vi "Generate Thetas.vi"(0 "spline flat":cluster{"x":sgl, "y":sgl}[](array[cluster]), 5 "starting angle":sgl, 7 "dt":sgl=0.02, 9 "ctrl pts":cluster{sgl, sgl}[][](array[cluster]), 11 "y unflat":cluster{dbl[]}[](array[cluster])) -> (4 "omega":sgl[](array[numeric]), 6 "theta":sgl[](array[numeric]), 10 "Tangent Vector":cluster{"x out":dbl, "y out":dbl}[](array[cluster]))   [LabVIEW 2025]
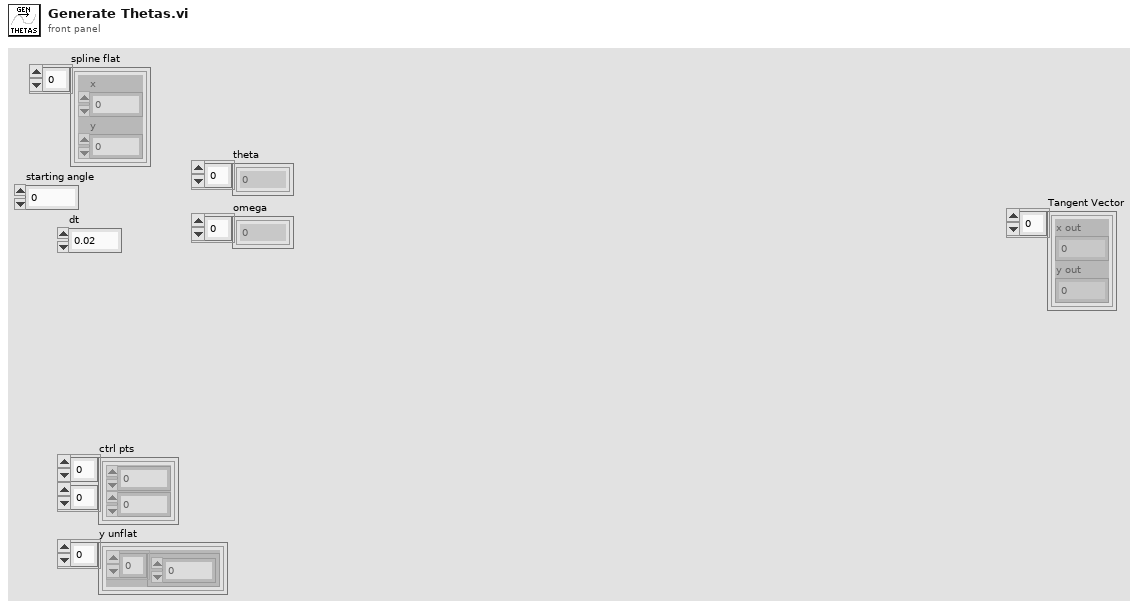
[diagram p1: front panel]
types:
  T1 = typedef "Bezier Curve.ctl" = cluster{"x":sgl, "y":sgl}[]
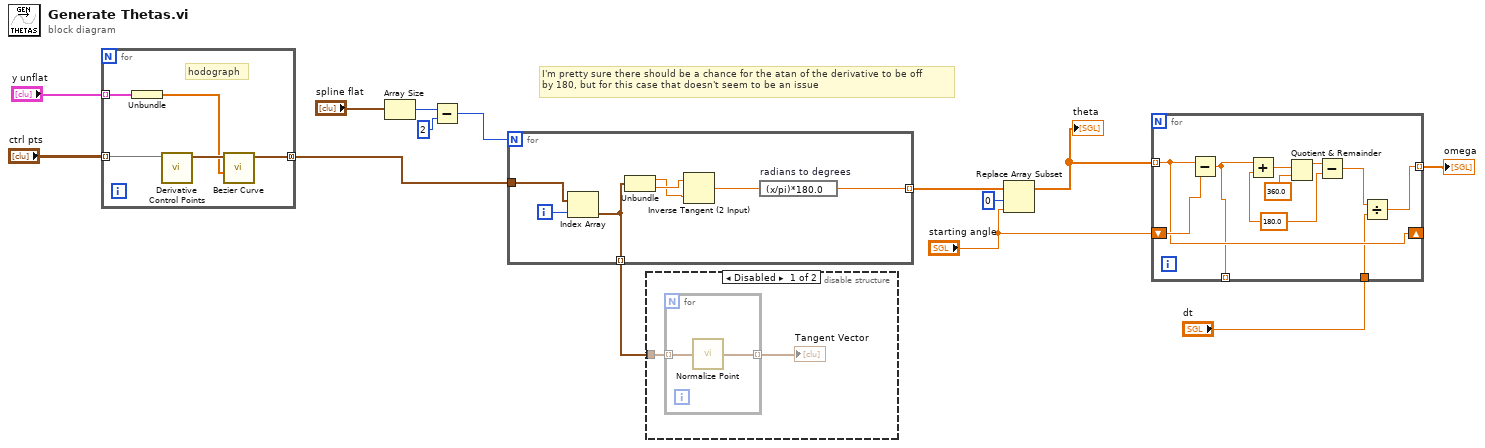
[diagram p0: block diagram]
diagram:
  # "I'm pretty sure there should be a chance for the atan of the derivative to be off\nby 180, but for this case that doesn't seem to be an issue"
  n1 = for {
    tunnel: "ctrl pts" -> [w19] mode=indexing
    tunnel: "y unflat" -> [w17] mode=indexing
    tunnel: [w15] -> w5 mode=concatenating
    # "hodograph"
    n2 = Unbundle(w17) -> (w16:dbl[])
    n3 = call "Derivative Control Points.vi"("ctrl points"=w19) -> ("d ctrl pts"=w18:cluster{dbl, dbl}[])  [unwired: 10 in]
    n4 = call "Bezier Curve.vi"("position"=w16, "ctrl points"=w18) -> ("curve"=w15:T1)  [unwired: 8 in, 1 out]
  }
  n5 = Array Size(array="spline flat") -> (size(s)=w14:i32)
  n6 = Subtract(x=w14, y=2) -> (x-y=w12:i32)
  n7 = for {
    N: w12 -> [_]
    tunnel: w5 -> [w22]
    tunnel: [w23] -> w11 mode=indexing
    tunnel: [w20] -> w1 mode=indexing
    i -> [w21]
    n8 = Index Array(array=w22, index=w21) -> (element=w20:cluster{"x":sgl, "y":sgl})
    n9 = Unbundle(w20) -> ("x"=w25:sgl, "y"=w26:sgl)
    n10 = Inverse Tangent (2 Input)(1:w25, 2:w26) -> (0:w24:sgl)
    n11 = expression code="(x/pi)*180.0" "radians to degrees"(w24) -> (w23:sgl)
  }
  n12 = disable-structure shown="Disabled" {
    disable-tunnel: w1 -> [w28 _]
    frame Disabled {
      n13 = for {
        tunnel: w28 -> [w29] mode=indexing
        tunnel: [w30] -> w27 mode=indexing
        n14 = call "Normalize Point.vi"("point in"=w29) -> ("point out"=w30:cluster{"x":sgl, "y":sgl})
      }
      "Tangent Vector" <- w27
    }
    frame Enabled {
    }
  }
  n15 = Replace Array Subset(array=w11, new element="starting angle", index=0) -> (w2:sgl[])
  "theta" <- w2
  n16 = for {
    tunnel: w2 -> [w39] mode=indexing
    shift-right: [w39] -> _
    shift-left: "starting angle" -> [w40]
    tunnel: [w37] -> w8 mode=indexing
    tunnel: "dt" -> [w38]
    tunnel: [w36] -> _ mode=indexing
    w31 = sgl 180.0 ("y")
    n17 = Subtract(x=w39, y=w40) -> (x-y=w36:sgl)
    n18 = Add(x=w36, y=w31) -> (x+y=w35:sgl)
    n19 = Quotient & Remainder(x=w35, y=sgl 360.0) -> (x-y*floor(x/y)=w32:sgl)  [unwired: 1 out]
    n20 = Subtract(x=w32, y=w31) -> (x-y=w33:sgl)
    n21 = Divide(x=w33, y=w38) -> (x/y=w37:sgl)
  }
  "omega" <- w8
